vi "Navi Distance Traveled Calc.vi"(0 "Right Avg":dbl, 1 "Left Avg":dbl, 2 "Reset X Y":dbl, 4 "Shift Register 1 In":dbl, 5 "Shift Register 2 In":dbl, 6 "Shift Register 3 In":dbl, 7 "Shift Register 4 In":dbl, 8 "Start X":dbl, 10 "Start Y":dbl) -> (16 "Right Side Setpoint":dbl, 18 "Left Side Setpoint":dbl, 20 "X Position":dbl, 21 "Y Position":dbl, 22 "Distance Traveled":dbl, 24 "Shift register 1 Out":dbl format="%#_13g", 25 "Shift register 2 Out":dbl format="%#_13g", 26 "Shift register 3 Out":dbl format="%#_13g", 27 "Shift register 4 Out":dbl format="%#_13g")   [LabVIEW 2015]
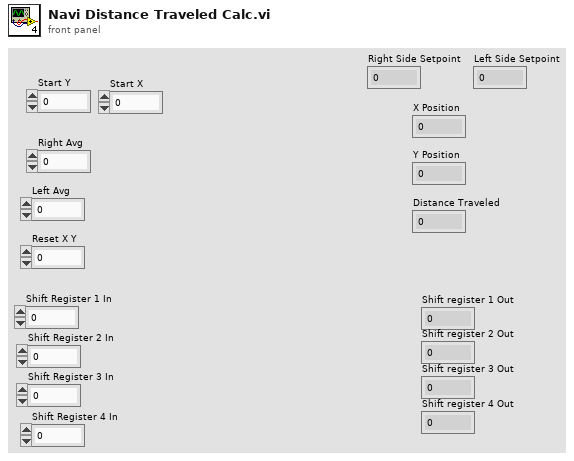
[diagram p1: front panel]
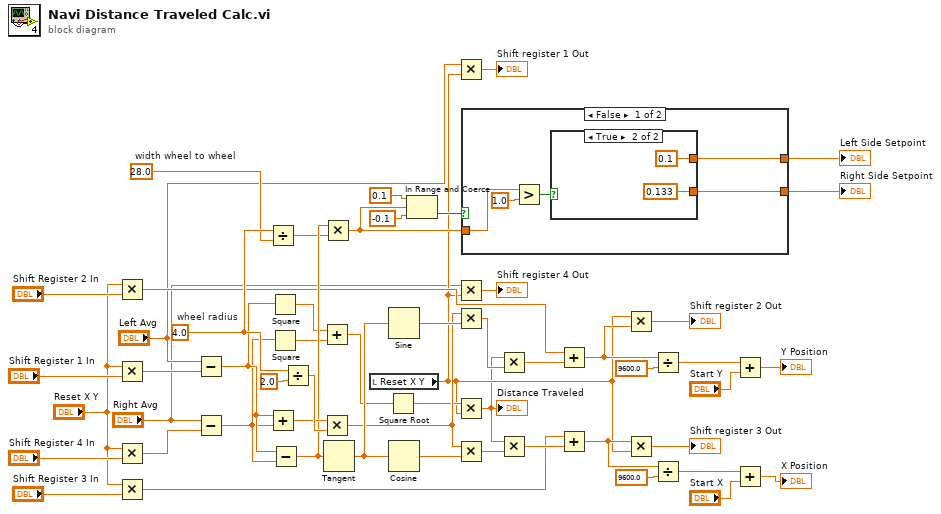
[diagram p0: block diagram]
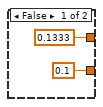
[diagram p2: hidden frame]
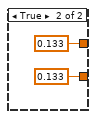
[diagram p3: hidden frame]
diagram:
  w44 = 28.0  # width wheel to wheel
  w45 = 4.0  # wheel radius
  n1 = Multiply(x="Reset X Y", y="Shift Register 2 In") -> (x*y=w18:dbl)
  n2 = Multiply(x="Reset X Y", y="Shift Register 1 In") -> (x*y=w19:dbl)
  n3 = Multiply(x="Reset X Y", y="Shift Register 4 In") -> (x*y=w16:dbl)
  n4 = Multiply(x="Reset X Y", y="Shift Register 3 In") -> (x*y=w17:dbl)
  n5 = Subtract(x="Left Avg", y=w19) -> (x-y=w38:dbl)
  n6 = Subtract(x="Right Avg", y=w16) -> (x-y=w37:dbl)
  n7 = Divide(x=w45, y=w44) -> (x/y=w40:dbl)
  n8 = Add(x=w38, y=w37) -> (x+y=w42:dbl)
  n9 = Square(x=w38) -> (x^2=w35:dbl)
  n10 = Square(x=w37) -> (x^2=w36:dbl)
  n11 = Subtract(x=w38, y=w37) -> (x-y=w41:dbl)
  n12 = Divide(x=w45, y=2.0) -> (x/y=w43:dbl)
  n13 = Add(x=w35, y=w36) -> (x+y=w34:dbl)
  n14 = Multiply(x=w42, y=w43) -> (x*y=w31:dbl)
  n15 = Multiply(x=w41, y=w40) -> (x*y=w12:dbl)
  n16 = Tangent(1:w41) -> (0:w39:dbl)
  n17 = local read "Reset X Y"() -> (w10:dbl)
  n18 = Square Root(x=w34) -> (sqrt(x)=w28:dbl)
  n19 = Sine(x=w39) -> (sin(x)=w33:dbl)
  n20 = Cosine(x=w39) -> (cos(x)=w32:dbl)
  n21 = In Range and Coerce(upper limit=0.1, x=w12, lower limit=-0.1) -> (In Range?=w13:bool)  [unwired: 1 out]
  n22 = Multiply(x="Left Avg", y=w10) -> (x*y=→"Shift register 1 Out":dbl)
  n23 = Multiply(x="Right Avg", y=w10) -> (x*y=→"Shift register 4 Out":dbl)
  n24 = Multiply(x=w31, y=w33) -> (x*y=w30:dbl)
  n25 = Multiply(x=w28, y=w10) -> (x*y=w5:dbl)
  "Distance Traveled" <- w5
  n26 = Multiply(x=w31, y=w32) -> (x*y=w29:dbl)
  n27 = case shown="False" w13 {
    tunnel: w12 -> [w59 _]
    tunnel: [w56 0.133] -> w2
    tunnel: [w55 0.133] -> w1
    frame False {
      n28 = Greater?(x=w59, y=1.0) -> (0:w57:bool)
      n29 = case shown="True" w57 {
        tunnel: [0.1333 0.1] -> w56
        tunnel: [0.1 0.133] -> w55
        frame False {
        }
        frame True {
        }
      }
    }
    frame True {
    }
  }
  "Left Side Setpoint" <- w2
  "Right Side Setpoint" <- w1
  n30 = Multiply(x=w5, y=w30) -> (x*y=w26:dbl)
  n31 = Multiply(x=w5, y=w29) -> (x*y=w27:dbl)
  n32 = Add(x=w18, y=w26) -> (x+y=w21:dbl)
  n33 = Add(x=w17, y=w27) -> (x+y=w25:dbl)
  n34 = Multiply(x=w10, y=w21) -> (x*y=→"Shift register 2 Out":dbl)
  n35 = Multiply(x=w25, y=w10) -> (x*y=→"Shift register 3 Out":dbl)
  n36 = Divide(x=w21, y=9600.0) -> (x/y=w23:dbl)
  n37 = Divide(x=w25, y=9600.0) -> (x/y=w22:dbl)
  n38 = Add(x=w23, y="Start Y") -> (x+y=→"Y Position":dbl)
  n39 = Add(x=w22, y="Start X") -> (x+y=→"X Position":dbl)
